vi "Store and Publish Device.vi"(8 "error in (no error)":errorcluster, 10 "Device":refnum<class "Device.lvclass">, 11 "picoG in":refnum<class "picoG.lvclass">) -> (0 "error out":errorcluster, 3 "picoG out":refnum<class "picoG.lvclass">)   [LabVIEW 2020, in "PicoG-App.lvlib" / "picoG.lvclass"]
uses:
  picoG.lvclass
  DeviceListPanel/DeviceListPanel.lvclass
  Device/Device.lvclass
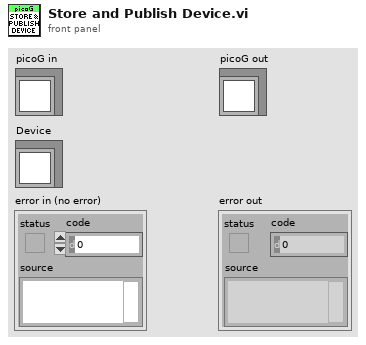
[diagram p1: front panel]
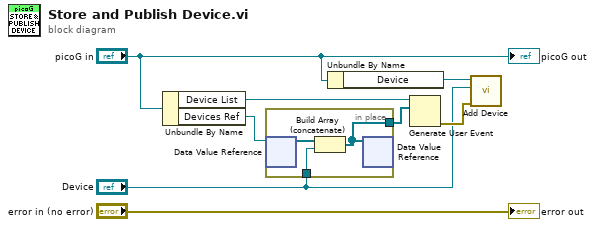
[diagram p0: block diagram]
diagram:
  n1 = Unbundle By Name("picoG in") -> ("Device List"=w3:refnum<user-event>, "Devices Ref"=w5:refnum<data-value>)
  n2 = in-place {
    in-place-border: "Device" -> [w10]
    in-place-border: [w9] -> w2
    n3 = in-place-dvr #1(w5) -> (w11:refnum<class "Device.lvclass">[])  [unwired: 1 out]
    n4 = Build Array (concatenate)(w11, w10) -> (w9:refnum<class "Device.lvclass">[])
    n5 = in-place-dvr #1(w9) -> ()  [unwired: 2 out]
  }
  n6 = Unbundle By Name("picoG in") -> ("Device"=w6:refnum<class "DeviceListPanel.lvclass">)
  n7 = Generate User Event(user event=w3, event data cluster=w2) -> (error out=w8:errorcluster)  [unwired: 2 in, 1 out]
  n8 = call "Add Device.vi"("error in (no error)"=w8, "Device"="Device", "DeviceListPanel in"=w6) -> ()  [unwired: 7 in, 2 out]
  "error out" <- "error in (no error)"
  "picoG out" <- "picoG in"
